vi "Distance Drive.vi"(4 "omni?":bool, 6 "reinit?":bool, 7 "PID Params":T1={"X Dist"={"PID gains"={"proportional gain (Kc)"=1.0, "integral time (Ti, min)"=0.0, "derivative time (Td, min)"=0.0}, "output range"={"output high"=1.0, "output low"=-1.0}}, "Y Dist"={"PID gains"={"proportional gain (Kc)"=1.0, "integral time (Ti, min)"=0.0, "derivative time (Td, min)"=0.0}, "output range"={"output high"=1.0, "output low"=-1.0}}} {"Y Dist"."output range"."output low" format="%.2f"; "Y Dist"."output range"."output high" format="%.2f"; "Y Dist"."PID gains"."derivative time (Td, min)" format="%.3f"; "Y Dist"."PID gains"."integral time (Ti, min)" format="%.3f"; "Y Dist"."PID gains"."proportional gain (Kc)" format="%.3f"; "X Dist"."output range"."output low" format="%.2f"; "X Dist"."output range"."output high" format="%.2f"; "X Dist"."PID gains"."derivative time (Td, min)" format="%.3f"; "X Dist"."PID gains"."integral time (Ti, min)" format="%.3f"; "X Dist"."PID gains"."proportional gain (Kc)" format="%.3f"}, 8 "distance target":cluster{"x":dbl, "y":dbl}, 9 "coast?":bool, 10 "Heading":dbl) -> (0 "X":dbl, 1 "Y":dbl, 3 "X steer":dbl)   [LabVIEW 2013]
uses:
  Distance Drive Result.ctl
  Common Code/Change Detect Boolean.vi
  Common Code/Change Detect Double.vi
  Robot Global Data.vi
panel:
  out "isFinished":bool
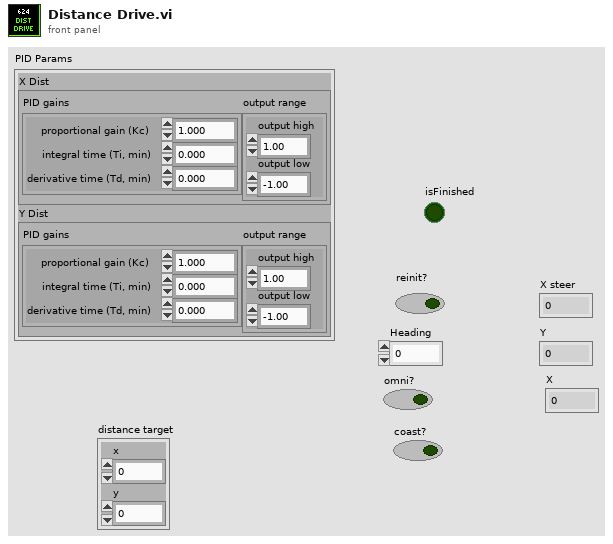
[diagram p1: front panel]
types:
  T1 = cluster{"X Dist":cluster{"PID gains":cluster{"proportional gain (Kc)":dbl, "integral time (Ti, min)":dbl, "derivative time (Td, min)":dbl}, "output range":cluster{"output high":dbl, "output low":dbl}}, "Y Dist":cluster{"PID gains":cluster{"proportional gain (Kc)":dbl, "integral time (Ti, min)":dbl, "derivative time (Td, min)":dbl}, "output range":cluster{"output high":dbl, "output low":dbl}}}
  T2 = typedef "Distance Drive Result.ctl" = cluster{"Finished":bool, "distance target":cluster{"x":dbl, "y":dbl}, "Heading Target":dbl, "X Check":bool, "Y Check":bool, "X Dist":dbl, "Y Dist":dbl}
  T3 = typedef "Dashboard UDP Packet.ctl" = cluster{"Camera":T4, "Gyro":T5, "Encoder":T7, "Auto Shift":T8, "Auton":T9, "Drive/Ramp X":dbl, "Drive/Ramp Y":dbl, "Drive/Battery Cutoff":dbl, "Pressure/Compressor Min Voltage":dbl, "Pressure/Compressor Delay":dbl, "Controller/Strafe Correction":bool, "Shooter":T10, "Rollers":T11, "Abort":bool, "Finish":bool}
  T4 = typedef "Camera Controls.ctl" = cluster{"Camera/View Angle X":dbl, "Camera/Goal Track Timeout":dbl, "Camera/View Angle Y":dbl, "Camera/Goal Exposure":dbl, "Camera/Vision Receive Timeout":dbl, "Camera/Offset 1":dbl, "Camera/Offset 2":dbl}
  T5 = typedef "Gyro Controls.ctl" = cluster{"Gyro/Angle Tolerance":dbl, "Gyro/Steer Closeness Threshold":dbl, "Steer PID":T6, "Steer Close PID":T6}
  T6 = typedef "PID Params.ctl" = cluster{"max":dbl, "min":dbl, "P":dbl, "I":dbl, "D":dbl}
  T7 = typedef "Encoder Controls.ctl" = cluster{"Encoders/Reset":bool, "Encoders/Omni Constant":dbl, "Encoders/Omni Tick Constant":dbl, "Encoders/Left Constant":dbl, "Encoders/Right Constant":dbl, "Encoders/Right Tick Constant":dbl}
  T8 = typedef "Auto Shift Controls.ctl" = cluster{"AutoShift/Upshift Throttle Accel":dbl, "AutoShift/Speed Threshold":dbl, "AutoShift/Upshift Throttle":dbl, "AutoShift/Upshift Accel":dbl, "AutoShift/Downshift Accel":dbl, "AutoShift/Downshift Throttle":dbl, "AutoShift/Delay":dbl, "AutoShift/Enabled":bool}
  T9 = typedef "Auton Controls.ctl" = cluster{"Auton/Left Shoot X-Coord":dbl, "Auton/Right Shoot X-Coord":dbl, "DistDrive/Distance Stop Threshold":dbl, "DistDrive/Max Stop Speed":dbl, "Auton/Back Piston Time":dbl, "Auton/Manual Hot":bool, "Auton/Manual Hot Right":bool, "Default X PID":T6, "Default Y PID":T6}
  T10 = typedef "Shooter Controls.ctl" = cluster{"Shooter/Reset Time":dbl, "Shooter/Release Delay":dbl, "Shooter/Pressure Steady Time":dbl, "Shooter/Misfire Delay":dbl, "Shooter/Ball Settle Time":dbl, "Shooter/Line IR Delay":dbl, "Pressure/Upper PSI Time":dbl, "Pressure/Lower PSI Time":dbl, "Shooter/Punch Delay":dbl, "Shooter/Target Pressure":dbl, "Pressure/Line B":dbl, "Pressure/Line M":dbl, "Pressure/Shooter M":dbl, "Pressure/Shooter B":dbl}
  T11 = typedef "Roller Controls.ctl" = cluster{"Roller/Load IRs Verify Time":dbl, "Roller/Center IR Latch Time":dbl, "Roller/Speed Front":dbl, "Roller/Speed Back":dbl, "Roller/Entry Timeout":dbl, "Roller/To Center Timeout":dbl, "Roller/Sustain Time":dbl, "Roller/Verify Center Time":dbl}
  T12 = typedef "Encoder Data.ctl" = cluster{"Avg Distance L/R":dbl, "Avg Speed L/R":dbl, "Left":T13, "Right":T13, "Omni":T13}
  T13 = typedef "Single Encoder Data.ctl" = cluster{"Distance":dbl, "Speed":dbl, "Ticks":dbl}
  T14 = cluster{"PID gains":cluster{"proportional gain (Kc)":dbl, "integral time (Ti, min)":dbl, "derivative time (Td, min)":dbl}, "output range":cluster{"output high":dbl, "output low":dbl}}
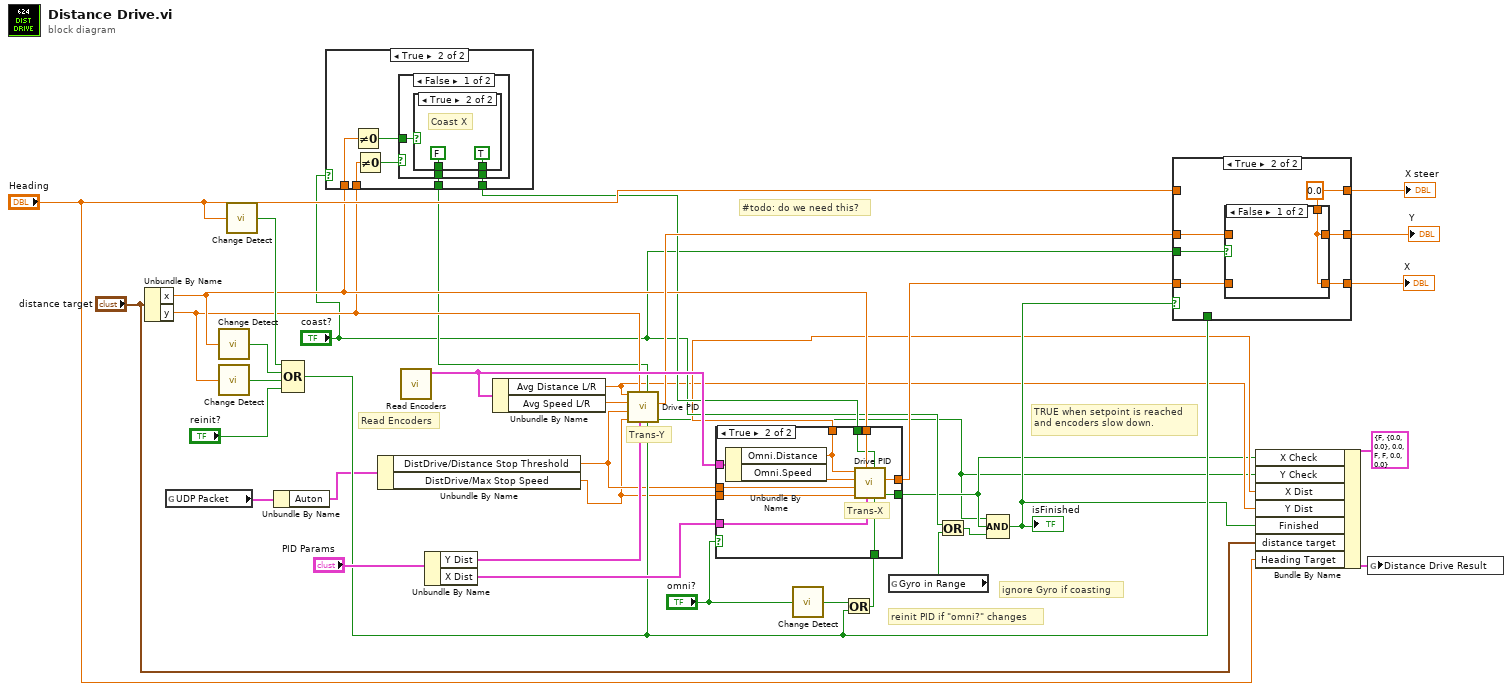
[diagram p0: block diagram]
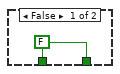
[diagram p2: hidden frame]
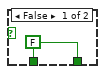
[diagram p3: hidden frame]
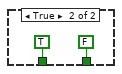
[diagram p4: hidden frame]
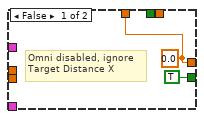
[diagram p5: hidden frame]
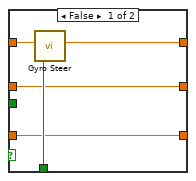
[diagram p6: hidden frame]
diagram:
  # "ignore Gyro if coasting"
  # "reinit PID if \"omni?\" changes"
  # "#todo: do we need this?"
  # "Trans-Y"
  # "Read Encoders"
  # "TRUE when setpoint is reached\nand encoders slow down."
  n1 = Unbundle By Name("distance target") -> ("x"=w15:dbl, "y"=w14:dbl)
  n2 = global read "Robot Global Data.vi" "UDP Packet"() -> (w8:T3)
  n3 = call-poly "Change Detect.vi"("In"=w15) -> ("Changed?"=w25:bool)
  n4 = call-poly "Change Detect.vi"("In"=w14) -> ("Changed?"=w24:bool)
  n5 = call-poly "Change Detect.vi"("In"="Heading") -> ("Changed?"=w21:bool)
  n6 = Unbundle By Name(w8) -> ("Auton"=w7:T9)
  n7 = Compound Arithmetic op=OR(w21, w25, w24, "reinit?") -> (w22:bool)
  n8 = case shown="True" "coast?" {
    tunnel: w15 -> [_ w45]
    tunnel: w14 -> [_ w44]
    tunnel: [w39 w41] -> w13
    tunnel: [w39 w40] -> w12
    frame False {
      w39 = FALSE
    }
    frame True {
      n9 = Not Equal To 0?(x=w45) -> (x != 0?=w42:bool)
      n10 = Not Equal To 0?(x=w44) -> (x != 0?=w43:bool)
      n11 = case shown="False" w43 {
        tunnel: w42 -> [w48 _]
        tunnel: [w47 FALSE] -> w41
        tunnel: [w46 TRUE] -> w40
        frame False {
          n12 = case shown="True" w48 {
            tunnel: [w49 TRUE] -> w47
            tunnel: [w49 FALSE] -> w46
            frame False {
              w49 = FALSE
            }
            frame True {
              # "Coast X"
            }
          }
        }
        frame True {
        }
      }
    }
  }
  n13 = Unbundle By Name(w7) -> ("DistDrive/Distance Stop Threshold"=w6:dbl, "DistDrive/Max Stop Speed"=w5:dbl)
  n14 = call "Read Encoders.vi"() -> ("Encoder Data"=w32:T12)  [unwired: 11 in]
  n15 = Unbundle By Name("PID Params") -> ("Y Dist"=w35:T14, "X Dist"=w33:T14)
  n16 = Unbundle By Name(w32) -> ("Avg Distance L/R"=w3:dbl, "Avg Speed L/R"=w34:dbl)
  n17 = call "Drive PID.vi"("reinitialize? (F)"=w22, "coast?"=w12, "PID Params"=w35, "Setpoint"=w14, "Max Stop Speed"=w5, "Distance Stop Threshold"=w6, "Current Speed"=w34, "Current Distance"=w3) -> ("Finished"=w1:bool, "output"=w26:dbl)  [unwired: 2 in]
  n18 = call-poly "Change Detect.vi"("In"="omni?") -> ("Changed?"=w29:bool)
  n19 = Or(x=w29, y=w22) -> (x .or. y?=w28:bool)
  n20 = case shown="True" "omni?" {
    tunnel: w33 -> [_ w66]
    tunnel: w5 -> [_ w65]
    tunnel: w6 -> [_ w64]
    tunnel: w32 -> [_ w63]
    tunnel: [w54 w61] -> w30
    tunnel: [TRUE ("Finished") w60] -> w2
    tunnel: w15 -> [_ w59]
    tunnel: w28 -> [_ w58]
    tunnel: [w54 w57] -> w4
    tunnel: w13 -> [_ w56]
    frame False {
      w54 = 0.0 ("output")
      # "Omni disabled, ignore\nTarget Distance X"
    }
    frame True {
      # "Trans-X"
      n21 = Unbundle By Name(w63) -> ("Omni.Distance"=w57:dbl, "Omni.Speed"=w62:dbl)
      n22 = call "Drive PID.vi"("reinitialize? (F)"=w58, "coast?"=w56, "PID Params"=w66, "Setpoint"=w59, "Max Stop Speed"=w65, "Distance Stop Threshold"=w64, "Current Speed"=w62, "Current Distance"=w57) -> ("Finished"=w60:bool, "output"=w61:dbl)  [unwired: 2 in]
    }
  }
  n23 = global read "Robot Global Data.vi" "Gyro in Range"() -> (w10:bool)
  n24 = Or(x="coast?", y=w10) -> (x .or. y?=w11:bool)
  n25 = Compound Arithmetic op=AND(w1, w2, w11) -> (w18:bool)
  "isFinished" <- w18
  n26 = case shown="True" w18 {
    tunnel: "Heading" -> [w71 _]
    tunnel: w22 -> [w70 _]
    tunnel: w26 -> [w68 w75]
    tunnel: [w69 w72] -> w38
    tunnel: [w68 w76] -> w37
    tunnel: [w67 w74] -> w31
    tunnel: w30 -> [w67 w73]
    tunnel: "coast?" -> [_ w77]
    frame False {
      n27 = call "Gyro Steer.vi"("reinitialize? (F)"=w70, "Target Angle"=w71) -> ("Steering Out"=w69:dbl)  [unwired: 8 in, 1 out]
    }
    frame True {
      w72 = 0.0 ("Steering Out")
      n28 = case shown="False" w77 {
        tunnel: [w78 w80] -> w76
        tunnel: w75 -> [_ w80]
        tunnel: [w78 w79] -> w74
        tunnel: w73 -> [_ w79]
        tunnel: w72 -> [w78 _]
        frame False {
        }
        frame True {
          # "keep coasting"
        }
      }
    }
  }
  "X steer" <- w38
  "Y" <- w37
  "X" <- w31
  n29 = Bundle By Name(cluster=T2 {"Finished"=FALSE, "distance target"={"x"=0.0, "y"=0.0}, "Heading Target"=0.0, "X Check"=FALSE, "Y Check"=FALSE, "X Dist"=0.0, "Y Dist"=0.0} ("Distance Drive Result"), "X Check"=w2, "Y Check"=w1, "X Dist"=w4, "Y Dist"=w3, "Finished"=w18, "distance target"="distance target", "Heading Target"="Heading") -> (w19:T2)
  n30 = global write "Robot Global Data.vi" "Distance Drive Result"(w19) -> ()
